vi "有效值计算.vi"(1 "数组":i32[](array[numeric]), 2 "选项卡数值":enum32{"单体电压", "单体温度", "单体内阻", "单体SOC"}(ring)) -> (0 "有效位":bool[](array[boolean]))   [LabVIEW 2013]
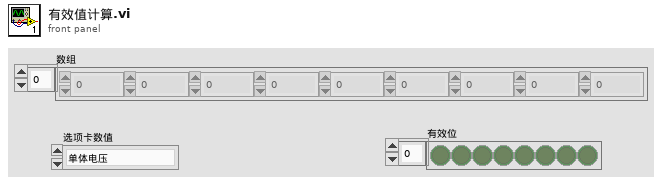
[diagram p1: front panel]
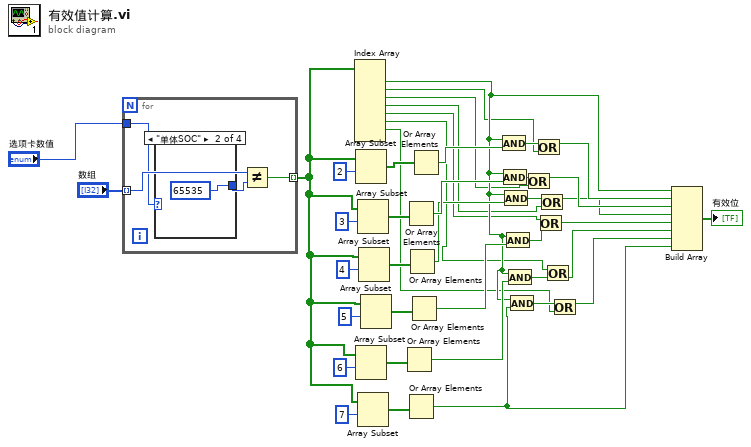
[diagram p0: block diagram]
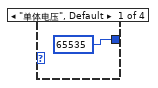
[diagram p2: hidden frame]
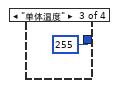
[diagram p3: hidden frame]
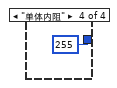
[diagram p4: hidden frame]
diagram:
  n1 = for {
    tunnel: "数组" -> [w44] mode=indexing
    tunnel: [w43] -> w18 mode=indexing
    tunnel: "选项卡数值" -> [w42]
    n2 = case shown="\"单体SOC\"" w42 {
      tunnel: [u16 65535 ("y") u16 65535 ("y") u16 255 ("y") u16 255 ("y")] -> w45
      frame "单体电压", Default {
      }
      frame "单体SOC" {
      }
      frame "单体温度" {
      }
      frame "单体内阻" {
      }
    }
    n3 = Not Equal?(x=w44, y=w45) -> (x != y?=w43:bool)
  }
  n4 = Index Array(array=w18) -> (element #1=w17:bool, element #2=w12:bool, element #3=w10:bool, element #4=w8:bool, element #5=w6:bool, element #6=w4:bool, element #7=w2:bool)  [unwired: 8 in, 1 out]
  n5 = Array Subset(array=w18, index=2 ("索引")) -> (w38:bool[])  [unwired: 1 in]
  n6 = Array Subset(array=w18, index=6 ("索引")) -> (w22:bool[])  [unwired: 1 in]
  n7 = Array Subset(array=w18, index=3 ("索引")) -> (w35:bool[])  [unwired: 1 in]
  n8 = Array Subset(array=w18, index=7 ("索引")) -> (w25:bool[])  [unwired: 1 in]
  n9 = Array Subset(array=w18, index=4 ("索引")) -> (w32:bool[])  [unwired: 1 in]
  n10 = Array Subset(array=w18, index=5 ("索引")) -> (w27:bool[])  [unwired: 1 in]
  n11 = Or Array Elements(Boolean array=w22) -> (logical OR=w19:bool)
  n12 = Or Array Elements(Boolean array=w35) -> (logical OR=w34:bool)
  n13 = Or Array Elements(Boolean array=w25) -> (logical OR=w15:bool)
  n14 = Or Array Elements(Boolean array=w32) -> (logical OR=w30:bool)
  n15 = Or Array Elements(Boolean array=w27) -> (logical OR=w26:bool)
  n16 = Or Array Elements(Boolean array=w38) -> (logical OR=w37:bool)
  n17 = And(x=w17, y=w37) -> (x .and. y?=w41:bool)
  n18 = And(x=w17, y=w34) -> (x .and. y?=w33:bool)
  n19 = And(x=w17, y=w30) -> (x .and. y?=w29:bool)
  n20 = And(x=w17, y=w26) -> (x .and. y?=w21:bool)
  n21 = And(x=w17, y=w19) -> (x .and. y?=w20:bool)
  n22 = And(x=w17, y=w15) -> (x .and. y?=w16:bool)
  n23 = Or(x=w33, y=w10) -> (x .or. y?=w11:bool)
  n24 = Or(x=w41, y=w12) -> (x .or. y?=w13:bool)
  n25 = Or(x=w6, y=w21) -> (x .or. y?=w7:bool)
  n26 = Or(x=w29, y=w8) -> (x .or. y?=w9:bool)
  n27 = Or(x=w4, y=w20) -> (x .or. y?=w5:bool)
  n28 = Or(x=w16, y=w2) -> (x .or. y?=w3:bool)
  n29 = Build Array(w17, w13, w11, w9, w7, w5, w3, w15) -> (→"有效位":bool[])
